vi "Dashboard Main1920x1080fixed_ALT.vi"() -> ()   [LabVIEW 2025]
uses:
  <vilib>/event_ctls.llb/eventvkey.ctl
  DashBoardGlobals.vi
  <vilib>/Rock Robotics/Network Tables/NT Read Numeric Array.vi
  <vilib>/Rock Robotics/WPI/Dashboard/WPI_DashboardLogging Global.vi
panel:
  in  "TCP":refnum<k5>
  out "NT Connection":bool
  out "Mode":T1(ring)=enum."Auto Disabled"
  out "BelowLeftCamBackground":bool
  out "Camera Perf":string
  in  "Rec Mode":enum32{"Stop", "Record", "Playback"}(radio)
  out "Robot IP":string
  in  "Dashboard Tab":T2(tab)
  out "MotorChart R":cluster{"Numeric":dbl, "Numeric":dbl}(graph)
  out "MotorChart L":cluster{"Numeric":dbl, "Numeric":dbl}(graph)
  out "MotorSliders R":cluster{"MotorSlide1":dbl, "MotorSlide2":dbl} {"MotorSlide2" scale=-1.0..1.0 scale format="%#_2e"; "MotorSlide1" scale=-1.0..1.0 scale format="%#_2e"}
  out "MotorSliders L":cluster{"MotorSlide1":dbl, "MotorSlide2":dbl} {"MotorSlide2" scale=-1.0..1.0 scale format="%#_2e"; "MotorSlide1" scale=-1.0..1.0 scale format="%#_2e"}
  out "JS1 Z":dbl(slide) scale=-1.0..1.0 scale format="%#_2e"
  out "JS1 Graph":cluster{"X":dbl, "Y":dbl}[](graph)
  out "JS1 Buttons":T3
  out "JS2 Z":dbl(slide) scale=-1.0..1.0 scale format="%#_2e"
  out "JS2 Graph":cluster{"X":dbl, "Y":dbl}[](graph)
  out "JS2 Buttons":T3
  out "Gyro":dbl(knob) scale=0.0..360.0
  in  "Update Agitator":bool
  in  "Agitator Desired Pct":dbl=1.0 min=-1.0 max=1.0 step=0.05 format="%8.2f"
  out "TurretLauncher/BallsLaunched":dbl caption="Balls Launched" format="%6.0f"
  out "Vision/Cam5Orientation":dbl caption="Cam 1 Yaw" format="%11.2f"
  out "Vision/Cam5Z":dbl caption="Cam 1 Z" format="%11.2f"
  out "Vision/Cam5Y":dbl caption="Cam 1 Y" format="%11.2f"
  out "Vision/Cam5Count":dbl caption="Cam1 Count" format="%13.0f"
  out "Vision/Cam5X":dbl caption="Cam 1 X" format="%11.2f"
  out "Vision/Cam4Orientation":dbl caption="Cam 1 Yaw" format="%11.2f"
  out "Vision/Cam4Z":dbl caption="Cam 1 Z" format="%11.2f"
  out "Vision/Cam4Y":dbl caption="Cam 1 Y" format="%11.2f"
  out "Vision/Cam4Count":dbl caption="Cam1 Count" format="%13.0f"
  out "Vision/Cam4X":dbl caption="Cam 1 X" format="%11.2f"
  out "Vision/Cam3Orientation":dbl caption="Cam 1 Yaw" format="%11.2f"
  out "Vision/Cam3Z":dbl caption="Cam 1 Z" format="%11.2f"
  out "Vision/Cam3Y":dbl caption="Cam 1 Y" format="%11.2f"
  out "Vision/Cam3Count":dbl caption="Cam1 Count" format="%13.0f"
  out "Vision/Cam3X":dbl caption="Cam 1 X" format="%11.2f"
  out "Vision/Cam2Orientation":dbl caption="Cam 1 Yaw" format="%11.2f"
  out "Vision/Cam2Z":dbl caption="Cam 1 Z" format="%11.2f"
  out "Vision/Cam2Y":dbl caption="Cam 1 Y" format="%11.2f"
  out "Vision/Cam2Count":dbl caption="Cam1 Count" format="%13.0f"
  out "Vision/Cam2X":dbl caption="Cam 1 X" format="%11.2f"
  out "Vision/Cam1Orientation":dbl caption="Cam 1 Yaw" format="%11.2f"
  out "Vision/Cam1Z":dbl caption="Cam 1 Z" format="%11.2f"
  out "Vision/Cam1Y":dbl caption="Cam 1 Y" format="%11.2f"
  out "Vision/Cam1Count":dbl caption="Cam1 Count" format="%13.0f"
  out "Vision/Cam1X":dbl caption="Cam 1 X" format="%11.2f"
  out "Climb/IsRetracted":bool caption="Retracted"
  out "Climb/MotorDemand":dbl caption="Pos Motor Dmd" format="%11.2f"
  out "Climb/Position":dbl caption="Position Act" format="%12.1f"
  out "Climb/RetractedLimitSwitch":bool caption="Retract Limit Switch"
  out "Climb/IsExtended":bool caption="Extended"
  out "AgitatorSystem/AgitatorStalled":bool caption="Agitator Stalled"
  out "AgitatorSystem/AgitatorRPMTarget":dbl caption="Speed Dmd  RPM" format="%12.1f"
  out "AgitatorSystem/AgitatorRPM":dbl caption="Speed  RPM" format="%12.1f"
  out "AgitatorSystem/AgitatorOutput":dbl caption="Motor Dmd" format="%11.2f"
  out "AgitatorSystem/AgitatorState":bool caption="Agitator On"
  out "IntakeSystem/BallMotorStalled":bool caption="Ball Intake Stalled"
  out "IntakeSystem/BallIntakeOn":bool caption="Ball Intake On"
  out "IntakeSystem/IntakeMotorRPM":dbl caption="Intake RPM" format="%12.1f"
  out "IntakeSystem/IntakeMotorOut":dbl caption="Intake Motor Dmd" format="%11.2f"
  out "TurretLauncher/TurretAngleVelocityDegSec":dbl caption="Pos Rate Deg/Sec" format="%12.1f"
  out "TurretLauncher/TurretManualMode":bool caption="Manual"
  out "TurretLauncher/TurretEncoderRotation":dbl caption="Pos Deg" format="%12.1f"
  out "TurretLauncher/TurretPositionOnTarget":bool caption="On Target"
  out "TurretLauncher/TurretMotorDmd":dbl caption="Motor Output" format="%11.2f"
  out "TurretLauncher/TurretDesiredAngle":dbl caption="Pos Dmd Deg" format="%12.1f"
  out "TurretLauncher/TurretclockwiseLimitSwitch":bool caption="CW Limit"
  out "TurretLauncher/TurretcounterclockwiseLimitSwitch":bool caption="CCW Limit"
  out "TurretLauncher/TurretDesiredAngleVel":dbl caption="Angle Velocity" format="%11.2f"
  out "TurretLauncher/TargetAngle":dbl caption="Angle" format="%11.2f"
  out "TurretLauncher/TargetDistance":dbl caption="Distance" format="%11.2f"
  out "FeederSystem/FeederTargetRPM":dbl caption="Speed Dnd RPM" format="%12.0f"
  out "FeederSystem/FeederRPM":dbl caption="Speed RPM" format="%12.0f"
  out "FeederSystem/FeederOutput":dbl caption="Motor Dmd" format="%11.2f"
  out "FeederSystem/FeederState":bool caption="Feeder On"
  out "MatchSystem/RobotCodePhase":T4(ring) caption="Code Phase"
  out "MatchSystem/isRed":bool caption="Is Red"
  out "MatchSystem/isBlue":bool caption="Is Blue"
  out "Supervisory/Mode":string caption="Mode"
  out "IntakeSystem/IntakeAngleMotorOut":dbl caption="Pos Motor Dmd" format="%11.2f"
  out "IntakeSystem/IntakeAngleTarget":dbl caption="Position Dmd Deg" format="%12.1f"
  out "IntakeSystem/IntakeAngleActual":dbl caption="Position Act Deg" format="%12.1f"
  out "IntakeSystem/IntakeLimitIsPressed":bool caption="LowLimitSwitch"
  out "IntakeSystem/IntakeIsExtended":bool caption="Extended"
  out "TurretLauncher/LauncherOn":bool caption="Launcher On"
  out "TurretLauncher/LauncherManualMode":bool caption="Manual"
  out "TurretLauncher/LauncherSpeed2":dbl caption="Motor 2 Speed" format="%11.0f"
  out "TurretLauncher/LauncherSpeed1":dbl caption="Motor 1 Speed" format="%11.0f"
  out "TurretLauncher/LauncherSpeedActual":dbl caption="Average Speed RPM" format="%11.0f"
  out "TurretLauncher/LauncherMotorDmd":dbl caption="Motor Dmd" format="%11.2f"
  out "TurretLauncher/LauncherTargetSpeed":dbl caption="Desired Speed RPM" format="%11.0f"
  out "TurretLauncher/LauncherSpeedOnTarget":bool caption="On Target"
  out "Teleop/GoClimb":bool caption="GO CLIMB"
  out "Teleop/FieldOriented":bool caption="Field Oriented"
  out "AutoSystem/StepTime":dbl caption="Step Time" format="%11.2f"
  out "Auto Selector":string caption="Name"
  out "AutoSystem/Step":T5(ring) caption="Cmd Name"
  out "AutoSystem/function":string caption="Function"
  out "AutoSystem/Parm2":dbl caption="Parm 2" format="%11.2f"
  out "AutoSystem/Parm1":dbl caption="Parm 1" format="%11.2f"
  out "AutoSystem/Timeout":dbl caption="Time out Sec" format="%11.2f"
  out "AutoSystem/Parm3":dbl caption="Parm 3" format="%11.2f"
  out "AutoSystem/Step":dbl caption="Cmd" format="%13.0f"
  out "TrajectorySystem/done":bool caption="Done"
  out "TrajectorySystem/ElapsedTrajTime":dbl caption="Elapsed Time" format="%12.1f"
  out "TrajectorySystem/rotErr":dbl caption="Rotational Error" format="%11.2f"
  out "TrajectorySystem/yErr":dbl caption="Y Error" format="%11.2f"
  out "TrajectorySystem/timeLengthOfTrajectory":dbl caption="Total Time" format="%12.1f"
  out "TrajectorySystem/xErr":dbl caption="X Error" format="%11.2f"
  out "TrajectorySystem/onTarget":bool caption="On Target"
  out "SwerveDrive/omegaActual":dbl caption="Vel Rot" format="%11.2f"
  out "SwerveDrive/vyActual":dbl caption="Vel Y" format="%12.1f"
  out "SwerveDrive/vyTarget":dbl caption="Vel Y Dmd" format="%12.1f"
  out "SwerveDrive/vxActual":dbl caption="Vel X" format="%12.1f"
  out "SwerveDrive/vxTarget":dbl caption="Vel X Dmd" format="%12.1f"
  out "SwerveDrive/GyroYaw":dbl caption="Gyro Yaw" format="%12.1f"
  out "SwerveDrive/GyroRoll":dbl caption="Gyro Roll" format="%12.1f"
  out "SwerveDrive/omegaTarget":dbl caption="Vel Rot Dmd" format="%11.2f"
  out "SwerveDrive/GyroPitch":dbl caption="Gyro Pitch" format="%12.1f"
  out "SwerveDrive/GyroConnected":bool caption="Gyro Connected"
  in  "Select Auto":string(combo)="Select Autonomous ..."
  out "Odometry/Rotation_position":dbl caption="Rotation Rad" format="%11.2f"
  out "Odometry/Y_position":dbl caption="Y Pos M" format="%11.2f"
  out "Odometry/execElapsedTime":dbl caption="Elapsed Time" format="%9.3f"
  out "Odometry/X_position":dbl caption="X Pos M" format="%11.2f"
  in  "Test Slider":dbl(slide) scale=0.0..100.0 scale format="%#_3g"
  in  "On/Off":bool caption="Solenoid"
  in  "Test Name":u16(ring) items=["Select the test to run..."]
  in  "Test Tree":string(tree)
  in  "Motor":cluster{"Value":dbl, "Enable":bool} {"Value" scale=-1.0..1.0 scale format="%#_3g"}
  out "Progress":T6 {"Test Progress" scale=0.0..100.0}
  in  "Rev/Fwd":cluster{"Forward":bool, "Reverse":bool}
  in  "Test Ring":u16(ring) items=["Monochrome", "Color"]
  in  "CheckList":i32(listbox)
  out "Tree":string(tree)
  out "Background":bool
  # "Drive Motors"
  # "Front"
  # "Right"
  # "Left"
  # "Back"
  # "Joysticks"
  # "TARGET"
  # "BALLS LAUNCHED"
  # "VISION"
  # "Cam 1"
  # "Cam 2"
  # "Cam 3"
  # "Cam 4"
  # "Cam 5"
  # "Count"
  # "X"
  # "Y"
  # "Z"
  # "Yaw"
  # "CLIMB"
  # "AGITATOR"
  # "BALL INTAKE"
  # "TURRET"
  # "FEEDER"
  # "MATCH"
  # "SUPERVISORY"
  # "INTAKE ARM"
  # "LAUNCHER"
  # "TELEOP"
  # "AUTO"
  # "TRAJECTORY"
  # "DRIVE"
  # "ODOMETRY"
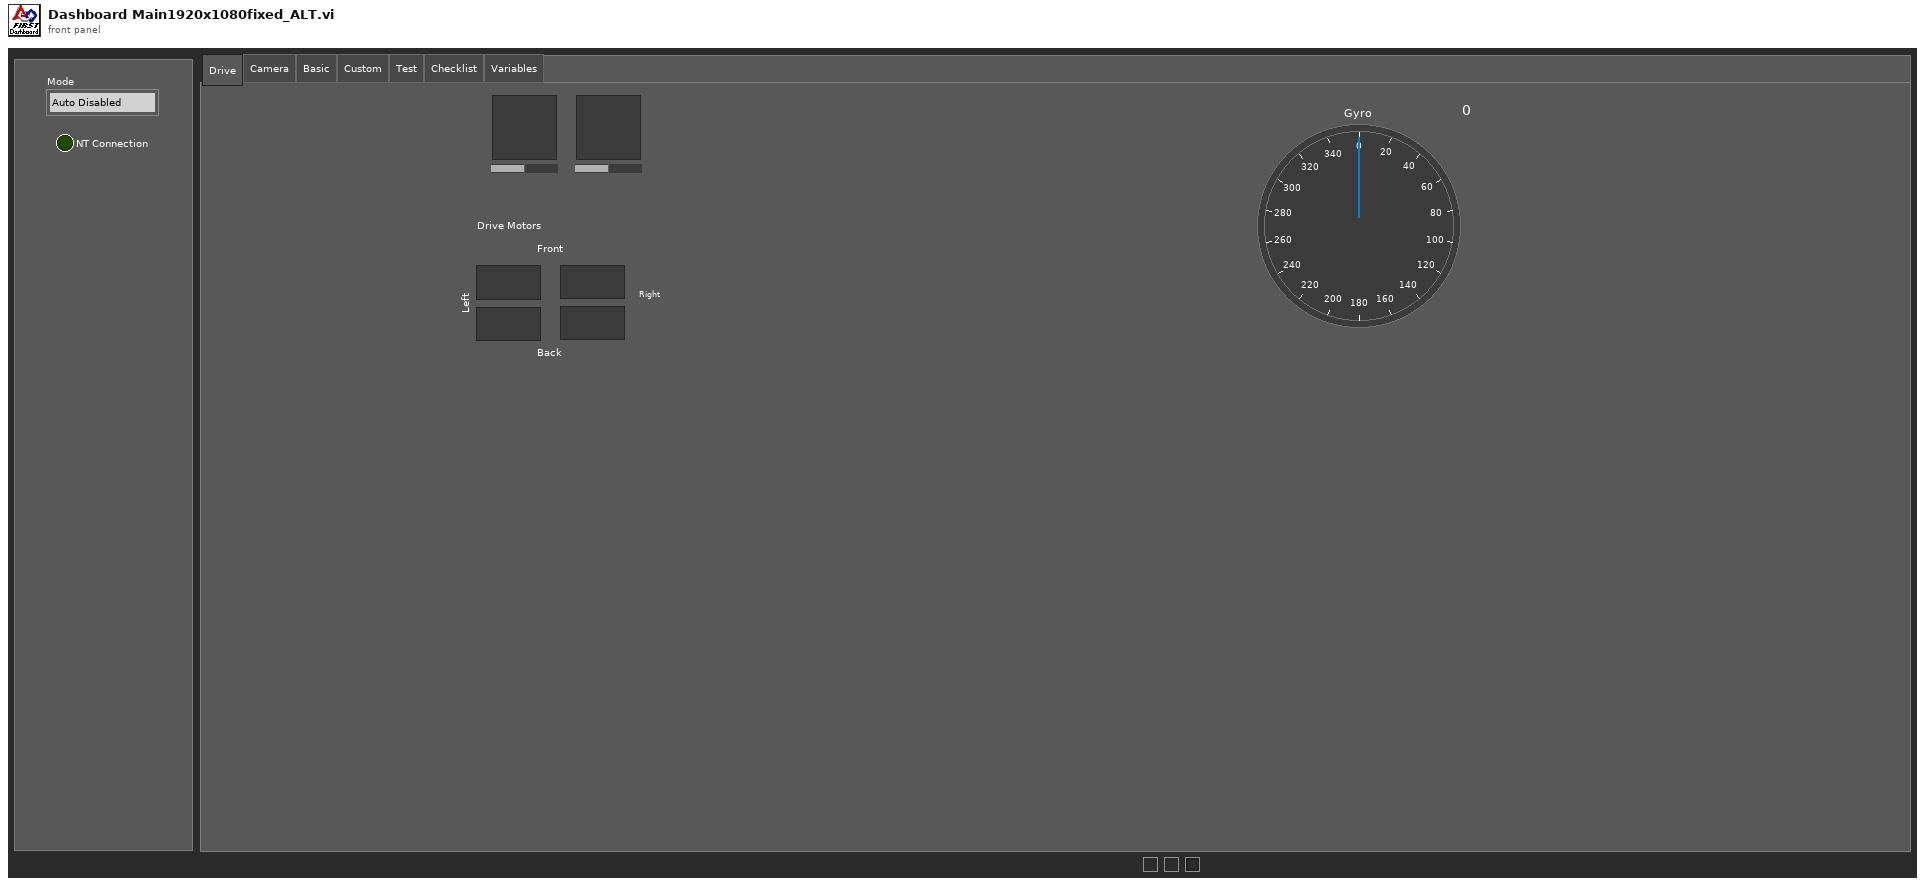
[diagram p1: front panel]
types:
  T1 = enum8{"Tele-Op Disabled", "Tele-Op Enabled", "Auto Disabled", "Auto Enabled", "Test Disabled", "Test Enabled", "Disconnected", "No Code", "E-Stop"}
  T2 = enum32{"Drive", "Camera", "Basic", "Custom", "Test", "Checklist", "Variables"}
  T3 = cluster{bool, bool, bool, bool, bool, bool, bool, bool, bool, bool, bool, bool}
  T4 = enum16{"Initial Startup", "Gyro Calibrated", "Trajectories Read", "Autos Read", "Startup Done", "Exec Disable Code", "Auto Init Done", "Auto Running", "Teleop Running"}
  T5 = enum16{"Drive Straight", "Drive Spin", "Follow Abs Traj", "Follow Rel Traj", "Wait", "Follow Abs Traj w/Event", "Follow Rel Traj w/Event", "Collect", "Shoot", "Balls To Alliance", "Climb", "Descend", "Unknown"}
  T6 = cluster{"Test Progress":u8, "Test Progress Text":string}
  T7 = enum32{"Invalid", "Standard", "Closed", "Hidden", "Minimized", "Maximized"}
  T8 = enum32{"Drive", "Camera", "Basic", "Custom", "Test", "Commands", "Checklist", "Variables"}
  T9 = cluster{"Error Strings":string, "Disable Counts":cluster{u16, u16}, "Rail Faults":cluster{u16, u16, u16}, "Robot IP":string, "DB Mode":u8, "Event Info":cluster{"Name":string, "Type":u8, "Number":u16, "Replay":u8}}
  T10 = cluster{"Storage":cluster{"Disk Free":u64, "RAM Block":u32, "RAM free":u32}, "CPU Utilization":cluster{"CPU % ISR":sgl, "CPU % Time Crit":sgl, "CPU % Timed Str":sgl, "CPU % High":sgl, "CPU % Above":sgl, "CPU % Normal":sgl, "CPU % Low":sgl}, "CAN":cluster{"% Bus Utilization":sgl, "Bus Off Cnt":u32, "TX_FIFO Full Cnt":u32, "Receive Error Cnt":u8, "Transmit Error Cnt":u8}, "HID":cluster{"HID Outputs":u32, "Rumble Low":u16, "Rumble High":u16}[]}
  T11 = cluster{"Status bits":cluster{"Test Mode":bool, "Autonomous":bool, "Enabled":bool, "Code Start":bool, "Brownout":bool, "Reserved 2":bool, "Reserved 3":bool, "E-Stop":bool}, "Code Trace":cluster{"Disabled":bool, "TeleOp":bool, "Auto":bool, "Test":bool}, "Controller Type":enum16{"unknown", "cRIO", "roboRio"}, "Code?":enum16{"unknown", "noCode", "code"}, "Battery V":dbl}
  T12 = cluster{"Control Bits":cluster{"TestMode":bool, "Autonomous":bool, "Enabled":bool, "FMS Present":bool, bool, bool, bool, "E-Stop":bool}, "Team Station ":u8, "Countdown":sgl, "Joystick Values":cluster{"Axes":dbl[], "Buttons":bool[], "POVs":i16[]}[]}
  T13 = cluster{"Axes":dbl[], "Buttons":bool[], "POVs":i16[]}[]
  T14 = cluster{"Axes":dbl[], "Buttons":bool[], "POVs":i16[]}
  T15 = cluster{"Buttons[0]":bool, "Buttons[1]":bool, "Buttons[2]":bool, "Buttons[3]":bool, "Buttons[4]":bool, "Buttons[5]":bool, "Buttons[6]":bool, "Buttons[7]":bool, "Buttons[8]":bool, "Buttons[9]":bool, "Buttons[10]":bool, "Buttons[11]":bool}
  T16 = cluster{"Dashboard Tab":refnum<vi>, "Background":refnum<vi>, "Rec Mode":refnum<vi>, "Test Slider":refnum<vi>, "On/Off ":refnum<vi>, "Test Ring":refnum<vi>, "Rev/Fwd":refnum<vi>, "Test Name":refnum<vi>, "Motor":refnum<vi>, "Progress":refnum<vi>, "CheckList":refnum<vi>, "Tree":refnum<vi>, "Test Tree":refnum<vi>, "Camera Perf":refnum<vi>}
  T17 = cluster{"Operation":enum16{"Update", "Clear"}, "Color Box":u32}[]
  T18 = typedef "eventvkey.ctl" = enum16{"ASCII", "Enter", "Return", "Shift", "Ctrl", "Alt", "Cmd", "Opt", "Caps", "NumLock", "Clear", "Break", "Up", "Down", "Left", "Right", "Insert", "Delete", "Home", "End", "PageUp", "PageDown", "Escape", "Help", "Pause", "ScrollLock", "F1", "F2", "F3", "F4", "F5", "F6", "F7", "F8", "F9", "F10", "F11", "F12", "F13", "F14", "F15", "F16", "F17", "F18", "F19", "F20", "F21", "F22", "F23", "F24", "Play", "VolumeUp", "VolumeDown", "Mute", "Two Byte Char"}
  T19 = cluster{"Image Size":bool, "Image Type":bool, "Pixel Value":bool, "ROI Information":bool, "Zoom Factor":bool}
  T20 = cluster{"Operation":enum16{"Update", "Clear"}, "Color Box":u32}
  T21 = cluster{"Shift":bool, "Ctrl":bool, "Alt":bool, "Cmd":bool, "Opt":bool}
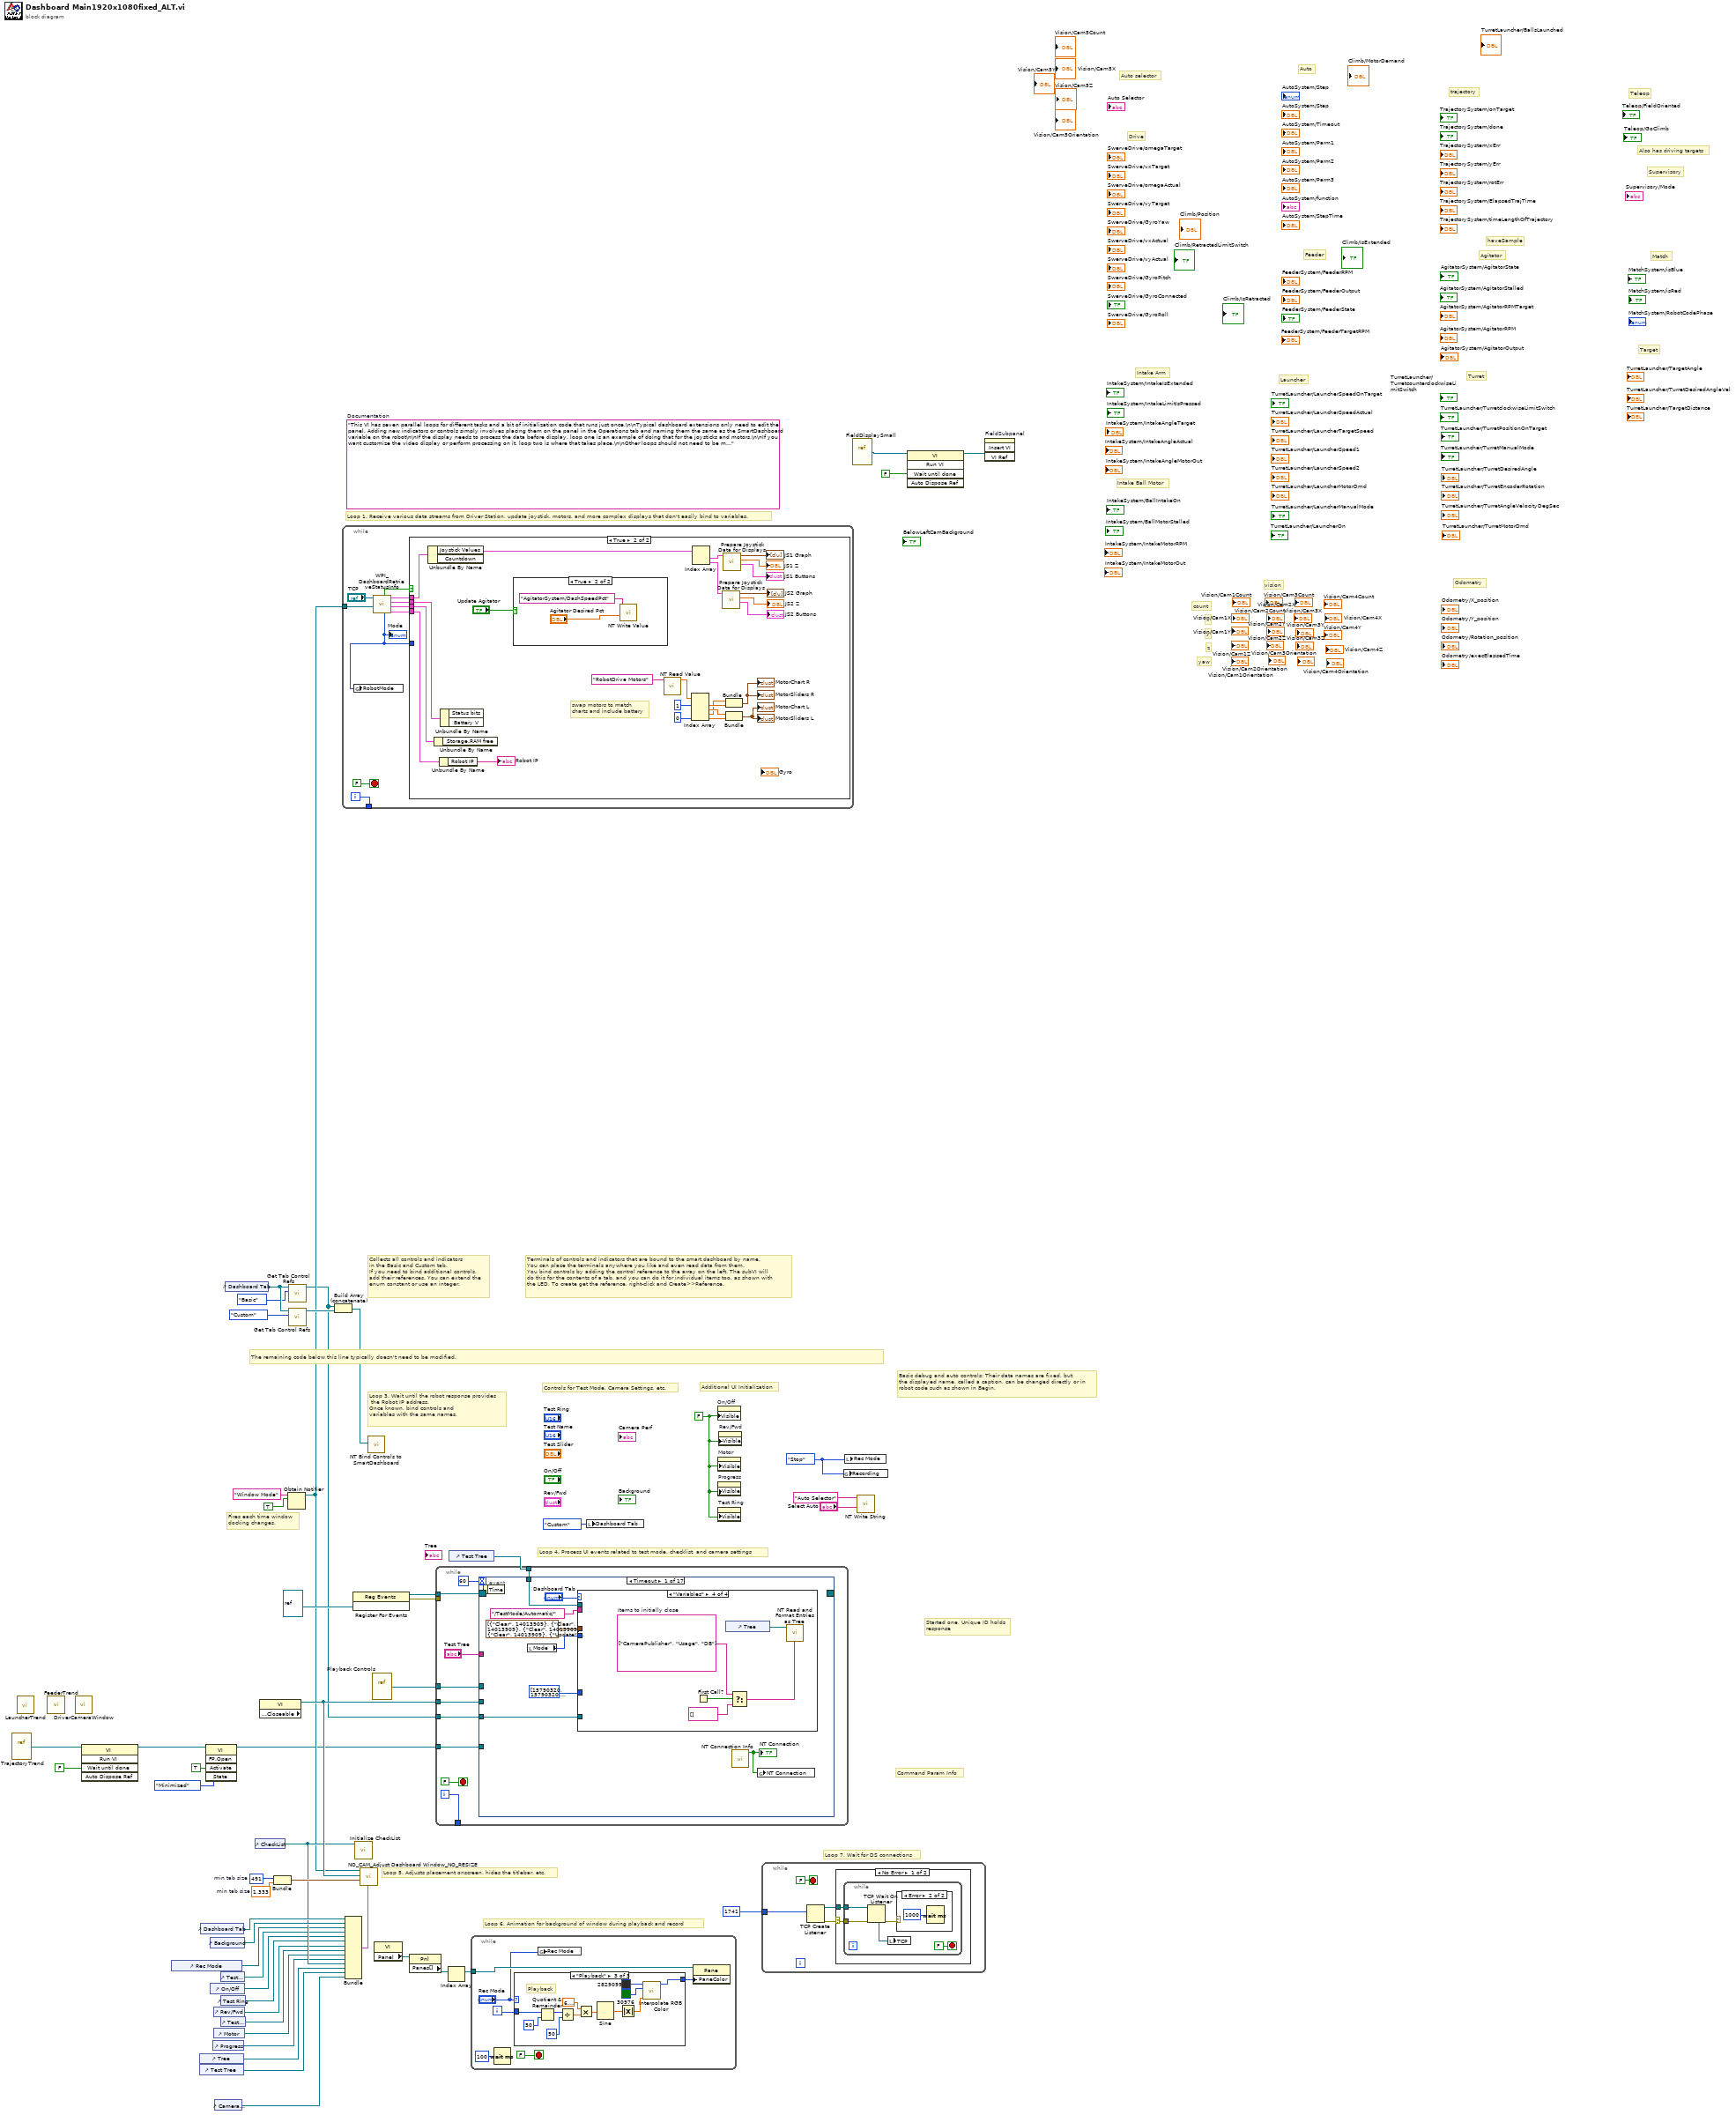
[diagram p0: block diagram]
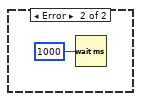
[diagram p3: hidden frame]
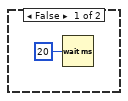
[diagram p4: hidden frame]
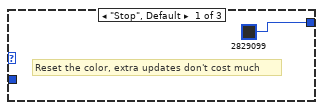
[diagram p6: hidden frame]
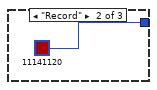
[diagram p7: hidden frame]
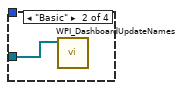
[diagram p9: hidden frame]
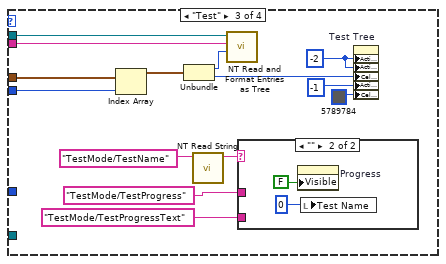
[diagram p10: hidden frame]
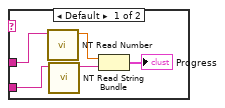
[diagram p11: hidden frame]
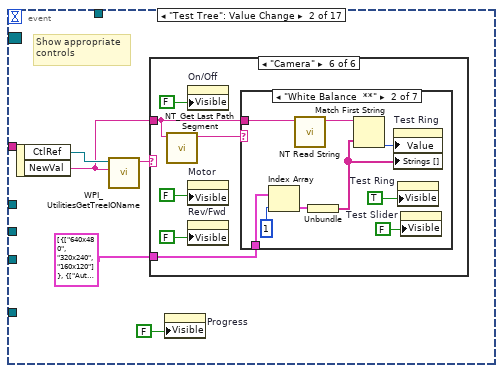
[diagram p12: hidden frame]
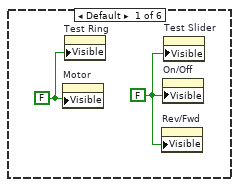
[diagram p13: hidden frame]
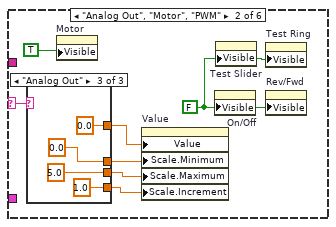
[diagram p14: hidden frame]
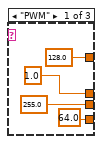
[diagram p15: hidden frame]
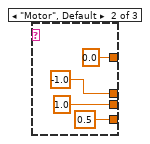
[diagram p16: hidden frame]
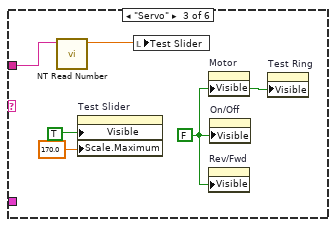
[diagram p17: hidden frame]
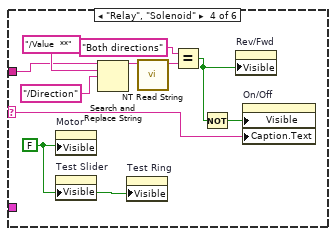
[diagram p18: hidden frame]
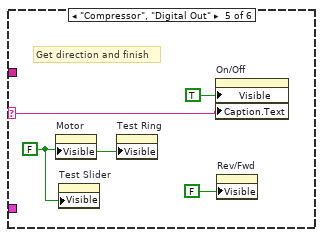
[diagram p19: hidden frame]
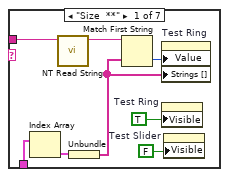
[diagram p20: hidden frame]
diagram:
  w35 = 491  # min tab size
  w34 = 1.333  # min tab size
  w41 = enum32{"Stop", "Record", "Playback"}."Stop" ("Rec Mode")
  w19 = FALSE ("Visible")
  (unwired) "This VI has seven parallel loops for different tasks and a bit of initialization code that runs just once.\n\nTypical dashboard extensions only need to edit the panel. Adding new indicators or controls simply involves placing them on the panel in the Operations tab and naming them the same as the SmartDashboard variable on the robot\n\nIf the display needs to process the data before display, loop one is an example of doing that for the joysticks and motors.\n\nIf you want customize the video display or perform processing on it, loop two is where that takes place.\n\nOther loops should not need to be modified. They are pretty standard, and document the task they perform."  # Documentation
  # "Intake Ball Motor"
  # "Target"
  # "Match"
  # "Supervisory"
  # "haveSample"
  # "Also has driving targets"
  # "Teleop"
  # "Odometry"
  # "Auto selector"
  # "Drive"
  # "Auto"
  # "trajectory"
  # "Feeder"
  # "Agitator"
  # "Intake Arm"
  # "Turret"
  # "yaw"
  # "z"
  # "y"
  # "x"
  # "count"
  # "vision"
  # "Launcher"
  # "Command Param Info"
  # "Started one, Unique ID holds\nresponse"
  # "Loop 7. Wait for DS connections"
  # "Basic debug and auto controls: Their data names are fixed, but\nthe displayed name, called a caption, can be changed directly or in\nrobot code such as shown in Begin."
  # "Controls for Test Mode, Camera Settings, etc."
  # "Additional UI Initialization"
  # "Loop 6. Animation for background of window during playback and record"
  # "Fires each time window\ndocking changes."
  # "Collects all controls and indicators\nin the Basic and Custom tab.\nIf you need to bind additional controls,\nadd their references. You can extend the\nenum constant or use an integer."
  # "The remaining code below this line typically doesn't need to be modified."
  # "Loop 4. Process UI events related to test mode, checklist, and camera settings"
  # "Terminals of controls and indicators that are bound to the smart dashboard by name.\nYou can place the terminals anywhere you like and even read data from them.\nYou bind controls by adding the control reference to the array on the left. The subVI will\ndo this for the contents of a tab, and you can do it for individual items too, as shown with\nthe LED. To create get the reference, right-click and Create>>Reference."
  # "Loop 3. Wait until the robot response provides\n the Robot IP address.\nOnce known, bind controls and\nvariables with the same names."
  # "Loop 5. Adjusts placement onscreen, hides the titlebar, etc."
  # "Loop 1. Receive various data streams from Driver Station, update joystick, motors, and more complex displays that don't easily bind to variables."
  n1 = vi-ref "TrajectoryTrend.vi"() -> (w5:refnum<vi>)
  n2 = call "LauncherTrend.vi"() -> ()  [unwired: 12 in]
  n3 = call "FeederTrend.vi"() -> ()  [unwired: 12 in]
  n4 = call "DriverCameraWindow.vi"() -> ()  [unwired: 1 in]
  n5 = invoke class="VI" method="Run VI"(reference=w5, "Wait until done"=FALSE ("Wait Until Done")) -> (reference out=w4:refnum<vi>)  [unwired: 3 in, 4 out]
  n6 = control-ref of="Rec Mode"() -> (w25:refnum<vi>)
  n7 = control-ref of="Tree"() -> (w29:refnum<vi>)
  n8 = control-ref of="Test Tree"() -> (w28:refnum<vi>)
  n9 = control-ref of="Dashboard Tab"() -> (w36:refnum<vi>)
  n10 = invoke class="VI" method="FP.Open"(reference=w4, "Activate"=TRUE ("Activate?"), "State"=T7."Minimized") -> (reference out=w1:refnum<vi>)  [unwired: 2 in, 4 out]
  n11 = control-ref of="Background"() -> (w32:refnum<vi>)
  n12 = control-ref of="On/Off"() -> (w23:refnum<vi>)
  n13 = control-ref of="Progress"() -> (w20:refnum<vi>)
  n14 = control-ref of="Rev/Fwd"() -> (w21:refnum<vi>)
  n15 = control-ref of="Motor"() -> (w26:refnum<vi>)
  n16 = control-ref of="Camera Perf"() -> (w16:refnum<vi>)
  n17 = control-ref of="Test Slider"() -> (w24:refnum<vi>)
  n18 = control-ref of="Test Ring"() -> (w22:refnum<vi>)
  n19 = control-ref of="Test Name"() -> (w27:refnum<vi>)
  n20 = control-ref of="Dashboard Tab"() -> (w39:refnum<vi>)
  n21 = control-ref of="CheckList"() -> (w30:refnum<vi>)
  n22 = property class="VI" props=["Front Panel.Closeable"]() -> (reference out=w40:refnum<vi>)  [unwired: 2 in, 2 out]
  n23 = Bundle("min tab size"=w35, "min tab size"=w34) -> (w33:cluster{"min tab size":i32, "min tab size":dbl})  [unwired: 1 in]
  n24 = Obtain Notifier(name (unnamed)="Window Mode", notification data type=TRUE) -> (notifier out=w18:refnum<notifier>)  [unwired: 2 in, 2 out]
  n25 = call <vilib>:"Get Tab Control Refs.vi"("Page Index"=T8."Basic" ("Dashboard Tab"), "TabControl in"=w39) -> ("ControlsOnPage"=w15:refnum<vi>[])  [unwired: 9 in]
  n26 = call <vilib>:"Get Tab Control Refs.vi"("Page Index"=T8."Custom" ("Dashboard Tab"), "TabControl in"=w39) -> ("ControlsOnPage"=w38:refnum<vi>[])  [unwired: 9 in]
  n27 = Build Array (concatenate)(w15, w38) -> (w37:refnum<vi>[])
  n28 = while {
    tunnel: [w60] -> _
    tunnel: w18 -> [w53]
    i -> [w60]
    stop <- FALSE stop-if-true
    n29 = call <vilib>:"WPI_DashboardRetrieveStatusInfo.vi"("Window Mode Notifier"=w53, "TCP Cnx"="TCP") -> ("Power and Errors"=w55:T9, "Robot Metrics"=w58:T10, "Status Info"=w59:T11, "Control Info"=w56:T12, "Robot Mode"=w52:T1, "Process?"=w57:bool)  [unwired: 4 in]
    "Mode" <- w52
    n30 = global write "DashBoardGlobals.vi" "RobotMode"(w52) -> ()
    n31 = case shown="True" w57 {
      tunnel: w59 -> [_ w87]
      tunnel: w58 -> [_ w86]
      tunnel: w56 -> [_ w85]
      tunnel: w55 -> [_ w84]
      tunnel: w52 -> [_ _]
      frame False {
        n32 = Wait (ms)(milliseconds to wait=u32 20) -> ()  [unwired: 1 out]
      }
      frame True {
        # "swap motors to match\ncharts and include battery"
        n33 = Unbundle By Name(w85) -> ("Joystick Values"=w75:T13)  [unwired: 1 out]
        n34 = Unbundle By Name(w86) -> ()  [unwired: 1 out]
        n35 = Unbundle By Name(w84) -> ("Robot IP"=→"Robot IP":string)
        n36 = Unbundle By Name(w87) -> ()  [unwired: 2 out]
        n37 = case shown="True" "Update Agitator" {
          frame False {
          }
          frame True {
            n38 = call-poly <vilib>:"NT Write Value.vi"("value"="Agitator Desired Pct", "name"="AgitatorSystem/DashSpeedPct") -> ()  [unwired: 9 in, 1 out]
          }
        }
        n39 = call-poly <vilib>:"NT Read Value.vi"("name"="RobotDrive Motors" ("Name")) -> ("value"=w65:dbl[])  [unwired: 8 in, 2 out]
        n40 = Index Array(array=w65, index #1=1, index #4=0) -> (element #1=w79:dbl, element #2=w80:dbl, element #3=w78:dbl, element #4=w83:dbl)  [unwired: 2 in]
        n41 = Index Array(array=w75) -> (element #1=w74:T14, element #2=w70:T14)  [unwired: 2 in]
        n42 = call "Prepare Joystick Data for Displays.vi"("Joystick Values"=w70) -> ("Buttons"=→"JS2 Buttons":T15, "Z Axis"=→"JS2 Z":dbl, "Cartesian Data"=→"JS2 Graph":cluster{"X axis":dbl, "X axis":dbl}[])  [unwired: 8 in]
        n43 = call "Prepare Joystick Data for Displays.vi"("Joystick Values"=w74) -> ("Buttons"=→"JS1 Buttons":T15, "Z Axis"=→"JS1 Z":dbl, "Cartesian Data"=→"JS1 Graph":cluster{"X axis":dbl, "X axis":dbl}[])  [unwired: 8 in]
        n44 = Bundle("Numeric"=w78, "Numeric"=w79) -> (→"MotorChart R" →"MotorSliders R":cluster{"Numeric":dbl, "Numeric":dbl})  [unwired: 1 in]
        n45 = Bundle("Numeric"=w80, "Numeric"=w83) -> (→"MotorChart L" →"MotorSliders L":cluster{"Numeric":dbl, "Numeric":dbl})  [unwired: 1 in]
      }
    }
  }
  n46 = Bundle("Dashboard Tab"=w36, "Background"=w32, "Rec Mode"=w25, "Test Slider"=w24, "On/Off"=w23, "Test Ring"=w22, "Rev/Fwd"=w21, "Test Name"=w27, "Motor"=w26, "Progress"=w20, "CheckList"=w30, "Tree"=w29, "Test Tree"=w28, "Camera Perf"=w16) -> (w31:T16)  [unwired: 1 in]
  n47 = register-events(refnum<vi> refnum) -> (reference out=w44:refnum<event-registration>, error out=w43:errorcluster)  [unwired: 2 in]
  n48 = call "Initialize CheckList.vi"("ListBox in"=w30) -> ()  [unwired: 11 in]
  n49 = call "NO_CAM_Adjust Dashboard Window_NO_RESIZE.vi"("Sizing Refnums"=w31, "Size Constraints"=w33, "VI"=w40, "WIn Mode"=w18) -> ()  [unwired: 8 in]
  n50 = call <vilib>:"NT Bind Controls to SmartDashboard.vi"("Bound Control Refs"=w37) -> ()  [unwired: 11 in]
  n51 = vi-ref "Playback Controls.vi"() -> (w45:refnum<vi>)
  n52 = property class="VI"() -> ("Panel"=w47:refnum<vi>)  [unwired: 2 in, 2 out]
  n53 = property class="Pnl"(reference=w47) -> ("Panes[]"=w48:refnum<vi>[])  [unwired: 1 in, 2 out]
  n54 = Index Array(array=w48) -> (element=w46:refnum<vi>)  [unwired: 1 in]
  n55 = control-ref of="Test Tree"() -> (w49:refnum<vi>)
  n56 = while {
    tunnel: [w96] -> _
    tunnel: w49 -> [w95]
    tunnel: w45 -> [w94]
    tunnel: w44 -> [w93]
    tunnel: w43 -> [_]
    tunnel: w40 -> [w92]
    tunnel: w15 -> [w91]
    tunnel: w1 -> [w90]
    i -> [w96]
    stop <- FALSE stop-if-true
    n57 = event shown="[0] Timeout" {
      selector: w93 -> [_ _ _ _ _ _ _ _ _ _ _ _ _ _ _ _ _]
      dyn-events: [_ _ _ _ _ _ _ _ _ _ _ _ _ w299 _ _ _] -> _
      timeout: u32 60 ("milliseconds to wait") -> [_ _ _ _ _ _ _ _ _ _ _ _ _ _ _ _ _]
      tunnel: w95 -> [w107 _ _ _ _ _ _ _ _ _ _ _ _ _ _ _ _]
      tunnel: "Test Tree" -> [_ _ _ _ _ _ _ _ w274 w281 w282 w285 w292 _ _ _ _]
      tunnel: w94 -> [_ _ _ _ _ _ _ _ _ _ _ _ _ w301 _ w319 _]
      tunnel: w92 -> [_ _ _ _ _ _ _ _ _ _ _ _ _ w297 _ _ _]
      tunnel: w91 -> [w102 _ _ _ _ _ _ _ _ _ _ _ _ _ _ _ _]
      tunnel: w90 -> [_ _ _ _ _ _ _ _ _ _ _ _ _ _ _ w314 _]
      event Timeout {
        n58 = event-data() -> ()  [unwired: 1 in, 1 out]
        n59 = local read "Mode"() -> (w105:T1)
        n60 = case shown="\"Variables\"" "Dashboard Tab" {
          tunnel: w107 -> [_ _ w122 _]
          tunnel: "/TestMode/Automatic/" ("Name Pattern") -> [_ _ w121 _]
          tunnel: T17 [{"Operation"=enum."Clear", "Color Box"=14013909}, {"Operation"=enum."Clear", "Color Box"=14013909}, {"Operation"=enum."Clear", "Color Box"=14013909}, {"Operation"=enum."Clear", "Color Box"=14013909}, {"Operation"=enum."Update", "Color Box"=14013909}, {"Operation"=enum."Update", "Color Box"=16777215}, {"Operation"=enum."Clear", "Color Box"=14013909}, {"Operation"=enum."Clear", "Color Box"=14013909}, {"Operation"=enum."Clear", "Color Box"=14013909}] -> [_ _ w114 _]
          tunnel: w105 -> [_ _ w113 _]
          tunnel: u32[] [15790320, 15790320, 15790320, 15790320, 16777215, 16777215, 15790320, 15790320, 15790320] -> [_ _ _ _]
          tunnel: w102 -> [_ w108 _ _]
          frame "Custom", Default {
          }
          frame "Basic" {
            n61 = call <vilib>:"WPI_DashboardUpdateNames.vi"("Controls on Tab"=w108) -> ()  [unwired: 11 in]
          }
          frame "Test" {
            w120 = -2 ("Active Item:Row Number")
            n62 = Index Array(array=w114, index=w113) -> (element=w115:T20)
            n63 = Unbundle(w115) -> ("Operation"=w116:enum16{"Update", "Clear"}, "Color Box"=w117:u32)
            n64 = call <vilib>:"NT Read String.vi"("name"="TestMode/TestName" ("Name")) -> ("value"=w111:string)  [unwired: 8 in, 2 out]
            n65 = call <vilib>:"NT Read and Format Entries as Tree.vi"("Operation"=w116, "Name Pattern"=w121, "Tree Refnum"=w122) -> ()  [unwired: 7 in, 2 out]
            n66 = case shown="\"\"" w111 {
              tunnel: "TestMode/TestProgress" ("Name") -> [w124 _]
              tunnel: "TestMode/TestProgressText" ("Name") -> [w123 _]
              frame Default {
                n67 = call <vilib>:"NT Read Number.vi"("name"=w124) -> ("value"=w125:dbl)  [unwired: 8 in, 2 out]
                n68 = call <vilib>:"NT Read String.vi"("name"=w123) -> ("value"=w126:string)  [unwired: 8 in, 2 out]
                n69 = Bundle("value"=w125, "value"=w126) -> (→"Progress":cluster{"value":dbl, "value":string})  [unwired: 1 in]
              }
              frame "" {
                n70 = property on="Progress" class="Clust (strict)"("Visible"=FALSE) -> ()  [unwired: 2 in, 2 out]
                n71 = local write "Test Name"(u16 0) -> ()
              }
            }
            n72 = property on="Test Tree" class="Tree (strict)"("Active Item Row Number"=w120, "ActiveColNum"=w120, "CellBG"=w117, "Active Item Row Number"=-1 ("Active Item:Row Number"), "CellBG"=u32 5789784 ("Color Box")) -> ()  [unwired: 2 in, 2 out]
          }
          frame "Variables" {
            w132 = string[] ["CameraPublisher", "Usage", "DB"]  # Items to initially close
            n73 = First Call?() -> (First Call?: T/F=w133:bool)
            n74 = control-ref of="Tree"() -> (w134:refnum<vi>)
            n75 = Select(t=w132, s=w133, f=string[] []) -> (s? t:f=w130:string[])
            n76 = call <vilib>:"NT Read and Format Entries as Tree.vi"("Tags to  Close"=w130, "Tree Refnum"=w134) -> ()  [unwired: 8 in, 2 out]
          }
        }
        n77 = call <vilib>:"NT Connection Info.vi"() -> ("Connected"=w100:bool)  [unwired: 11 in]
        "NT Connection" <- w100
        n78 = global write "DashBoardGlobals.vi" "NT Connection"(w100) -> ()
      }
      event "Test Tree": Value Change {
        # "Show appropriate\ncontrols"
        n79 = event-data() -> ("CtlRef"=w138:refnum<vi>, "NewVal"=w136:string)  [unwired: 1 in]
        n80 = call <vilib>:"WPI_UtilitiesGetTreeIOName.vi"("NewVal"=w136, "TreeControl in"=w138) -> ("I/O Name"=w139:string)  [unwired: 9 in]
        n81 = case shown="\"Camera\"" w139 {
          selector: w139 -> [_ w146 _ w168 w177 _]
          tunnel: w136 -> [_ _ w165 w167 _ w184]
          tunnel: cluster{string[]}[] [{["640x480", "320x240", "160x120"]}, {["Auto", "Fixed indoor", "Fixed outdoor 1", "Fixed outdoor 2", "Fixed fluorescent 1", "Fixed fluorescent 2", "Hold current"]}, {["Auto", "Flicker-free 50 Hz", "Flicker-free 60 Hz", "Hold current"]}, {["None", "Prioritize frame rate", "Prioritize image quality"]}, {["Monochrome", "Color"]}] -> [_ _ _ _ _ w183]
          frame Default {
            w141 = FALSE ("Visible")
            w140 = FALSE ("Visible")
            n82 = property on="Motor" class="Clust (strict)"("Visible"=w140) -> ()  [unwired: 2 in, 2 out]
            n83 = property on="Test Ring" class="Ring (strict)"("Visible"=w140) -> ()  [unwired: 2 in, 2 out]
            n84 = property on="Rev/Fwd" class="Clust (strict)"("Visible"=w141) -> ()  [unwired: 2 in, 2 out]
            n85 = property on="On/Off" class="Bool (strict)"("Visible"=w141) -> ()  [unwired: 2 in, 2 out]
            n86 = property on="Test Slider" class="Slide (strict)"("Visible"=w141) -> ()  [unwired: 2 in, 2 out]
          }
          frame "Analog Out", "Motor", "PWM" {
            w147 = FALSE ("Visible")
            n87 = case shown="\"Analog Out\"" w146 {
              tunnel: [1.0 ("Value") -1.0 ("Value") 0.0 ("Value")] -> w145
              tunnel: [255.0 ("Value") 1.0 ("Value") 5.0 ("Value")] -> w144
              tunnel: [128.0 ("Value") 0.0 ("Value") 0.0 ("Value")] -> w143
              tunnel: [64.0 ("Value") 0.5 ("Value") 1.0 ("Value")] -> w142
              frame "PWM" {
              }
              frame "Motor", Default {
              }
              frame "Analog Out" {
              }
            }
            n88 = property on="Motor" class="Clust (strict)"("Visible"=TRUE) -> ()  [unwired: 2 in, 2 out]
            n89 = property on="Value" class="Slide (strict)"("Value"=w143, "Scale.Minimum"=w145, "Scale.Maximum"=w144, "Scale.Increment"=w142) -> ()  [unwired: 2 in, 2 out]
            n90 = property on="On/Off" class="Bool (strict)"("Visible"=w147) -> ()  [unwired: 2 in, 2 out]
            n91 = property on="Test Slider" class="Slide (strict)"("Visible"=w147) -> ()  [unwired: 2 in, 2 out]
            n92 = property on="Test Ring" class="Ring (strict)"("Visible"=w147) -> ()  [unwired: 2 in, 2 out]
            n93 = property on="Rev/Fwd" class="Clust (strict)"("Visible"=w147) -> ()  [unwired: 2 in, 2 out]
          }
          frame "Servo" {
            w163 = FALSE ("Visible")
            n94 = call <vilib>:"NT Read Number.vi"("name"=w165) -> ("value"=w164:dbl)  [unwired: 8 in, 2 out]
            n95 = property on="Test Slider" class="Slide (strict)"("Visible"=TRUE, "Scale.Maximum"=170.0 ("Scale.Range:Maximum")) -> ()  [unwired: 2 in, 2 out]
            n96 = local write "Test Slider"(w164) -> ()
            n97 = property on="Motor" class="Clust (strict)"("Visible"=w163) -> ()  [unwired: 2 in, 2 out]
            n98 = property on="Rev/Fwd" class="Clust (strict)"("Visible"=w163) -> ()  [unwired: 2 in, 2 out]
            n99 = property on="On/Off" class="Bool (strict)"("Visible"=w163) -> ()  [unwired: 2 in, 2 out]
            n100 = property on="Test Ring" class="Ring (strict)"("Visible"=w163) -> ()  [unwired: 2 in, 2 out]
          }
          frame "Relay", "Solenoid" {
            w166 = FALSE ("Visible")
            n101 = property on="Motor" class="Clust (strict)"("Visible"=w166) -> ()  [unwired: 2 in, 2 out]
            n102 = property on="Test Slider" class="Slide (strict)"("Visible"=w166) -> ()  [unwired: 2 in, 2 out]
            n103 = Search and Replace String(input string=w167, search string="/Value  **", replace string="/Direction") -> (result string=w173:string)  [unwired: 5 in, 3 out]
            n104 = property on="Test Ring" class="Ring (strict)"("Visible"=w166) -> ()  [unwired: 2 in, 2 out]
            n105 = call <vilib>:"NT Read String.vi"("name"=w173) -> ("value"=w171:string)  [unwired: 8 in, 2 out]
            n106 = Equal?(x="Both directions", y=w171) -> (x = y?=w169:bool)
            n107 = Not(x=w169) -> (.not. x?=w170:bool)
            n108 = property on="Rev/Fwd" class="Clust (strict)"("Visible"=w169) -> ()  [unwired: 2 in, 2 out]
            n109 = property on="On/Off" class="Bool (strict)"("Visible"=w170, "Caption.Text"=w168) -> ()  [unwired: 2 in, 2 out]
          }
          frame "Compressor", "Digital Out" {
            w176 = FALSE ("Visible")
            # "Get direction and finish"
            n110 = property on="Motor" class="Clust (strict)"("Visible"=w176) -> ()  [unwired: 2 in, 2 out]
            n111 = property on="Test Slider" class="Slide (strict)"("Visible"=w176) -> ()  [unwired: 2 in, 2 out]
            n112 = property on="Test Ring" class="Ring (strict)"("Visible"=w176) -> ()  [unwired: 2 in, 2 out]
            n113 = property on="On/Off" class="Bool (strict)"("Visible"=TRUE, "Caption.Text"=w177) -> ()  [unwired: 2 in, 2 out]
            n114 = property on="Rev/Fwd" class="Clust (strict)"("Visible"=FALSE) -> ()  [unwired: 2 in, 2 out]
          }
          frame "Camera" {
            n115 = call <vilib>:"NT_Get Last Path Segment.vi"("String in"=w184) -> ("String out"=w185:string)  [unwired: 10 in]
            n116 = property on="On/Off" class="Bool (strict)"("Visible"=FALSE) -> ()  [unwired: 2 in, 2 out]
            n117 = property on="Motor" class="Clust (strict)"("Visible"=FALSE) -> ()  [unwired: 2 in, 2 out]
            n118 = property on="Rev/Fwd" class="Clust (strict)"("Visible"=FALSE) -> ()  [unwired: 2 in, 2 out]
            n119 = case shown="\"White Balance  **\"" w185 {
              tunnel: w184 -> [w191 w200 w209 w218 w227 _ w233]
              tunnel: w183 -> [w189 w197 w206 w215 w224 _ _]
              frame "Size  **" {
                n120 = Index Array(array=w189) -> (element=w188:cluster{string[]})  [unwired: 1 in]
                n121 = call <vilib>:"NT Read String.vi"("name"=w191) -> ("value"=w190:string)  [unwired: 8 in, 2 out]
                n122 = Unbundle(w188) -> (w186:string[])
                n123 = Match First String(2:w186, 3:w190) -> (0:w187:i32)  [unwired: 1 out]
                n124 = property on="Test Ring" class="Ring (strict)"("Value"=w187, "Strings []"=w186) -> ()  [unwired: 2 in, 2 out]
                n125 = property on="Test Ring" class="Ring (strict)"("Visible"=TRUE) -> ()  [unwired: 2 in, 2 out]
                n126 = property on="Test Slider" class="Slide (strict)"("Visible"=FALSE) -> ()  [unwired: 2 in, 2 out]
              }
              frame "White Balance  **" {
                n127 = Index Array(array=w197, index=1) -> (element=w198:cluster{string[]})
                n128 = call <vilib>:"NT Read String.vi"("name"=w200) -> ("value"=w199:string)  [unwired: 8 in, 2 out]
                n129 = Unbundle(w198) -> (w195:string[])
                n130 = Match First String(2:w195, 3:w199) -> (0:w194:i32)  [unwired: 1 out]
                n131 = property on="Test Ring" class="Ring (strict)"("Value"=w194, "Strings []"=w195) -> ()  [unwired: 2 in, 2 out]
                n132 = property on="Test Ring" class="Ring (strict)"("Visible"=TRUE) -> ()  [unwired: 2 in, 2 out]
                n133 = property on="Test Slider" class="Slide (strict)"("Visible"=FALSE) -> ()  [unwired: 2 in, 2 out]
              }
              frame "Exposure  **" {
                n134 = Index Array(array=w206, index=2) -> (element=w207:cluster{string[]})
                n135 = call <vilib>:"NT Read String.vi"("name"=w209) -> ("value"=w208:string)  [unwired: 8 in, 2 out]
                n136 = Unbundle(w207) -> (w203:string[])
                n137 = Match First String(2:w203, 3:w208) -> (0:w204:i32)  [unwired: 1 out]
                n138 = property on="Test Ring" class="Ring (strict)"("Value"=w204, "Strings []"=w203) -> ()  [unwired: 2 in, 2 out]
                n139 = property on="Test Ring" class="Ring (strict)"("Visible"=TRUE) -> ()  [unwired: 2 in, 2 out]
                n140 = property on="Test Slider" class="Slide (strict)"("Visible"=FALSE) -> ()  [unwired: 2 in, 2 out]
              }
              frame "Exposure Priority  **" {
                n141 = Index Array(array=w215, index=3) -> (element=w216:cluster{string[]})
                n142 = call <vilib>:"NT Read String.vi"("name"=w218) -> ("value"=w217:string)  [unwired: 8 in, 2 out]
                n143 = Unbundle(w216) -> (w212:string[])
                n144 = Match First String(2:w212, 3:w217) -> (0:w213:i32)  [unwired: 1 out]
                n145 = property on="Test Ring" class="Ring (strict)"("Value"=w213, "Strings []"=w212) -> ()  [unwired: 2 in, 2 out]
                n146 = property on="Test Ring" class="Ring (strict)"("Visible"=TRUE) -> ()  [unwired: 2 in, 2 out]
                n147 = property on="Test Slider" class="Slide (strict)"("Visible"=FALSE) -> ()  [unwired: 2 in, 2 out]
              }
              frame "Color Enable  **" {
                n148 = Index Array(array=w224, index=4) -> (element=w225:cluster{string[]})
                n149 = call <vilib>:"NT Read String.vi"("name"=w227) -> ("value"=w226:string)  [unwired: 8 in, 2 out]
                n150 = Unbundle(w225) -> (w221:string[])
                n151 = Match First String(2:w221, 3:w226) -> (0:w222:i32)  [unwired: 1 out]
                n152 = property on="Test Ring" class="Ring (strict)"("Value"=w222, "Strings []"=w221) -> ()  [unwired: 2 in, 2 out]
                n153 = property on="Test Ring" class="Ring (strict)"("Visible"=TRUE) -> ()  [unwired: 2 in, 2 out]
                n154 = property on="Test Slider" class="Slide (strict)"("Visible"=FALSE) -> ()  [unwired: 2 in, 2 out]
              }
              frame Default {
                n155 = property on="Test Ring" class="Ring (strict)"("Visible"=FALSE) -> ()  [unwired: 2 in, 2 out]
                n156 = property on="Test Slider" class="Slide (strict)"("Visible"=FALSE) -> ()  [unwired: 2 in, 2 out]
              }
              frame "Brightness  **", "Color Level  **", "Compression  **", "FPS  **", "Sharpness  **" {
                n157 = call <vilib>:"NT Read Number.vi"("name"=w233) -> ("value"=w232:dbl)  [unwired: 8 in, 2 out]
                n158 = local write "Test Slider"(w232) -> ()
                n159 = property on="Test Ring" class="Ring (strict)"("Visible"=FALSE) -> ()  [unwired: 2 in, 2 out]
                n160 = property on="Test Slider" class="Slide (strict)"("Visible"=TRUE, "Scale.Maximum"=100.0 ("Scale.Range:Maximum")) -> ()  [unwired: 2 in, 2 out]
              }
            }
          }
        }
        n161 = property on="Progress" class="Clust (strict)"("Visible"=FALSE) -> ()  [unwired: 2 in, 2 out]
      }
      event "Test Name": Mouse Enter {
        # "Populate the ring with the list of tests"
        n162 = event-data() -> ()  [unwired: 1 in, 1 out]
        n163 = call <vilib>:"NT Read String Array.vi"("name"="TestMode/TestList" ("Name")) -> ("value"=w240:string[])  [unwired: 8 in, 2 out]
        n164 = Build Array (concatenate)("Select the test to run...", w240) -> (w239:string[])
        n165 = property on="Test Name" class="Ring (strict)"("Strings []"=w239) -> ()  [unwired: 2 in, 2 out]
      }
      event "Test Name": Value Change {
        w241 = FALSE ("Visible")
        # "Tell the robot the test name to run"
        n166 = event-data() -> ("NewVal"=w245:u16)  [unwired: 1 in]
        n167 = property on="Test Name" class="Ring (strict)"() -> ("Strings []"=w246:string[])  [unwired: 2 in, 2 out]
        n168 = local write "Progress"(T6 {"Test Progress"=0, "Test Progress Text"=""} ("Progress")) -> ()
        n169 = Index Array(array=w246, index=w245) -> (element=w244:string)
        n170 = call <vilib>:"NT Write String.vi"("value"=w244, "name"="TestMode/TestName" ("Name")) -> ()  [unwired: 9 in, 1 out]
        n171 = property on="Progress" class="Clust (strict)"("Visible"=TRUE) -> ()  [unwired: 2 in, 2 out]
        n172 = property on="Motor" class="Clust (strict)"("Visible"=w241) -> ()  [unwired: 2 in, 2 out]
        n173 = property on="Test Slider" class="Slide (strict)"("Visible"=w241) -> ()  [unwired: 2 in, 2 out]
        n174 = property on="On/Off" class="Bool (strict)"("Visible"=w241) -> ()  [unwired: 2 in, 2 out]
        n175 = property on="Rev/Fwd" class="Clust (strict)"("Visible"=w241) -> ()  [unwired: 2 in, 2 out]
        n176 = property on="Test Ring" class="Ring (strict)"("Visible"=w241) -> ()  [unwired: 2 in, 2 out]
      }
      event "Select Auto": Mouse Enter {
        # "Populate the combo box with the list of autonomous options"
        n177 = event-data() -> ()  [unwired: 1 in, 1 out]
        n178 = call <vilib>:"NT Read String Array.vi"("name"="Auto List" ("Name")) -> ("value"=w248:string[])  [unwired: 8 in, 2 out]
        n179 = property on="Select Auto" class="CmbBox"("Strings[]"=w248) -> ()  [unwired: 2 in, 2 out]
      }
      event "Select Auto": Value Change {
        # "User modified the Auto Selection. Write to NT variable so robot knows."
        n180 = event-data() -> ("NewVal"=w250:string)  [unwired: 1 in]
        n181 = call <vilib>:"NT Write String.vi"("value"=w250, "name"="Auto Selector" ("Name")) -> ()  [unwired: 9 in, 1 out]
      }
      event "CheckList": Double Click {
        # "Shift clears all"
        # "Update symbols on the listbox"
        n182 = event-data() -> ("PlatMods.Shift"=w252:bool, "Row"=w254:i32)  [unwired: 1 in]
        n183 = case shown="True" w252 {
          tunnel: w254 -> [w258 _]
          tunnel: 1 -> [w257 _]
          frame False {
            n184 = property on="CheckList" class="LstBox (strict)"() -> ("Item Symbols"=w256:i32[])  [unwired: 2 in, 2 out]
            n185 = Replace Array Subset(array=w256, new element=w257, index=w258) -> (w255:i32[])
            n186 = property on="CheckList" class="LstBox (strict)"("Item Symbols"=w255) -> ()  [unwired: 2 in, 2 out]
          }
          frame True {
            w259 = 0 ("Top Row")
            n187 = property on="CheckList" class="LstBox (strict)"() -> ("Number of Rows"=w261:u32)  [unwired: 2 in, 2 out]
            n188 = Initialize Array(0, w261) -> (w260:i32[])
            n189 = property on="CheckList" class="LstBox (strict)"("Top Row"=w259, "Value"=w259, "Item Symbols"=w260) -> ()  [unwired: 2 in, 2 out]
          }
        }
      }
      event "CheckList": Key Down {
        # "Update symbols on the listbox\nLeft and right keys check and uncheck"
        n190 = event-data() -> ("VKey"=w264:T18)  [unwired: 1 in]
        n191 = case shown="\"Left\", \"Right\"" w264 {
          selector: w264 -> [w269 _]
          tunnel: eventvkey."Left" ("VKey") -> [w267 _]
          frame "Left", "Right" {
            n192 = Equal?(x=w267, y=w269) -> (x = y?=w268:bool)
            n193 = Select(t=0, s=w268, f=1) -> (s? t:f=w270:i32)
            n194 = property on="CheckList" class="LstBox (strict)"() -> ("Item Symbols"=w273:i32[])  [unwired: 2 in, 2 out]
            n195 = Replace Array Subset(array=w273, new element=w270, index="CheckList") -> (w272:i32[])
            n196 = property on="CheckList" class="LstBox (strict)"("Item Symbols"=w272) -> ()  [unwired: 2 in, 2 out]
          }
          frame Default {
          }
        }
      }
      event "Motor.Enable": Value Change {
        # "When the test mode otor enable helper is set, update that\ntree row item's value"
        n197 = event-data() -> ("NewVal"=w278:bool)  [unwired: 1 in]
        n198 = Unbundle("Motor") -> ("Value"=w277:dbl)  [unwired: 1 out]
        n199 = Select(t=w277, s=w278, f=0.0) -> (s? t:f=w275:dbl)
        n200 = call <vilib>:"NT Write Number.vi"("value"=w275, "name"=w274) -> ()  [unwired: 9 in, 1 out]
      }
      event "Test Slider": Value Change {
        # "When the test mode slider helper is set, update that\ntree row item's value"
        n201 = event-data() -> ("NewVal"=w280:dbl)  [unwired: 1 in]
        n202 = call <vilib>:"NT Write Number.vi"("value"=w280, "name"=w281) -> ()  [unwired: 9 in, 1 out]
      }
      event "On/Off": Value Change {
        # "When the test mode on/off helper value is set, update that\ntree row item's value"
        n203 = event-data() -> ("NewVal"=w284:bool)  [unwired: 1 in]
        n204 = Boolean To (0,1)(Boolean=w284) -> (0, 1=w283:i16)
        n205 = call <vilib>:"NT Write Number.vi"("value"=w283, "name"=w282) -> ()  [unwired: 9 in, 1 out]
      }
      event "Rev/Fwd": Value Change {
        # "When the test mode helper value for relays is set, update that\ntree row item's value"
        n206 = event-data() -> ("NewVal.Forward"=w291:bool, "NewVal.Reverse"=w290:bool)  [unwired: 1 in]
        n207 = Boolean To (0,1)(Boolean=w291) -> (0, 1=w287:i16)
        n208 = Boolean To (0,1)(Boolean=w290) -> (0, 1=w289:i16)
        n209 = Negate(x=w289) -> (-x=w288:i16)
        n210 = Add(x=w287, y=w288) -> (x+y=w286:i16)
        n211 = call <vilib>:"NT Write Number.vi"("value"=w286, "name"=w285) -> ()  [unwired: 9 in, 1 out]
      }
      event "Test Ring": Value Change {
        # "When a test mode helper value is selected from the ring,\nset the tree item's variable to the string value"
        n212 = event-data() -> ("NewVal"=w294:u16)  [unwired: 1 in]
        n213 = property on="Test Ring" class="Ring (strict)"() -> ("Strings []"=w295:string[])  [unwired: 2 in, 2 out]
        n214 = Index Array(array=w295, index=w294) -> (element=w293:string)
        n215 = call <vilib>:"NT Write String.vi"("value"=w293, "name"=w292) -> ()  [unwired: 9 in, 1 out]
      }
      event "Rec Mode": Value Change {
        # "Update globals for recording mode and path to read log from.\nClear when logging and let NetworkTables set path for vision to\nuse."
        n216 = event-data() -> ("NewVal"=w302:enum32{"Stop", "Record", "Playback"})  [unwired: 1 in]
        n217 = global write "WPI_DashboardLogging Global.vi" "Logging Filename"(path "") -> ()
        n218 = global write "WPI_DashboardLogging Global.vi" "Recording"(w302) -> ()
        n219 = case shown="\"Playback\"" w302 {
          tunnel: w301 -> [_ w304 w312]
          tunnel: [_ _ w311] -> w299
          tunnel: [_ _ w310] -> _
          tunnel: w297 -> [_ _ w308]
          tunnel: cluster{i32, i32} {-250, 170} -> [_ _ w307]
          tunnel: [_ _ T19 {"Image Size"=TRUE, "Image Type"=TRUE, "Pixel Value"=TRUE, "ROI Information"=TRUE, "Zoom Factor"=FALSE} ("Image Information Shown:All Elements")] -> _
          tunnel: [_ _ TRUE ("Zoom Factor")] -> _
          frame Default {
          }
          frame "Stop", "Record" {
            # "Place Window too"
            n220 = invoke class="VI" method="FP.Close"(reference=w304) -> (reference out=w303:refnum<vi>)  [unwired: 2 in, 2 out]
            n221 = invoke class="VI" method="Abort VI"(reference=w303) -> ()  [unwired: 2 in, 3 out]
          }
          frame "Playback" {
            n222 = call "Open Playback Panel.vi"("Offset"=w307, "DB VI Ref"=w308, "Playback in"=w312) -> ("Playback out"=w309:refnum<vi>)  [unwired: 8 in]
            n223 = register-events(w309) -> (reference out=w311:refnum<event-registration>, error out=w310:errorcluster)  [unwired: 2 in]
          }
        }
        n224 = call <vilib>:"WPI_DashboardNT Log FieldName Cache.vi"("Operation"=enum16{"Lookup/Add", "Index", "Clear"}."Clear") -> ()  [unwired: 8 in, 3 out]
      }
      event Panel Close {
        w313 = enum32{"Stop", "Record", "Playback"}."Stop" ("Rec Mode")
        # "Playback window has been closed, abort"
        n225 = event-data() -> ()  [unwired: 1 in, 4 out]
        n226 = local write "Rec Mode"(w313) -> ()
        n227 = global write "WPI_DashboardLogging Global.vi" "Recording"(w313) -> ()
      }
      event Panel Close {
        # "Abort playback window and ourself"
        n228 = event-data() -> ()  [unwired: 1 in, 4 out]
        n229 = invoke class="VI" method="FP.Close"(reference=w319) -> (reference out=w318:refnum<vi>)  [unwired: 2 in, 2 out]
        n230 = invoke class="VI" method="FP.Close"(reference=w314) -> (reference out=w316:refnum<vi>)  [unwired: 2 in, 2 out]
        n231 = invoke class="VI" method="Abort VI"(reference=w318) -> (error out=w317:errorcluster)  [unwired: 2 in, 2 out]
        n232 = invoke class="VI" method="Abort VI"(reference=w316) -> (error out=w315:errorcluster)  [unwired: 2 in, 2 out]
        n233 = invoke class="VI" method="Abort VI"(error in=w317) -> ()  [unwired: 2 in, 3 out]
        n234 = invoke class="VI" method="Abort VI"(error in=w315) -> ()  [unwired: 2 in, 3 out]
      }
      event "Tree": Double Click {
        n235 = event-data() -> ("PlatMods"=w325:T21, "Tag"=w322:string)  [unwired: 1 in]
        n236 = Unbundle(w325) -> ("Shift"=w324:bool)  [unwired: 4 out]
        n237 = String Subset(string=w322, length (rest)=1 ("length (rest)")) -> (substring=w321:string)  [unwired: 1 in]
        n238 = Not(x=w324) -> (.not. x?=w323:bool)
        n239 = case shown="\"/\"" w321 {
          tunnel: w322 -> [_ w327]
          tunnel: w323 -> [_ w326]
          frame Default {
          }
          frame "/" {
            n240 = call <vilib>:"NT Update Persistence.vi"("Persistence"=w326, "Name"=w327) -> ()  [unwired: 9 in, 1 out]
          }
        }
      }
    }
  }
  n241 = while {
    tunnel: w46 -> [w330]
    i -> [w332]
    stop <- FALSE stop-if-true
    n242 = Wait (ms)(milliseconds to wait=u32 100) -> ()  [unwired: 1 out]
    n243 = case shown="\"Playback\"" "Rec Mode" {
      tunnel: w332 -> [_ _ w347]
      tunnel: [u32 2829099 ("Base Color") u32 11141120 ("Target Color") w336] -> w329
      frame "Stop", Default {
        # "Reset the color, extra updates don't cost much"
      }
      frame "Record" {
      }
      frame "Playback" {
        # "Playback"
        n244 = Quotient & Remainder(x=w347, y=u32 50 ("milliseconds to wait")) -> (x-y*floor(x/y)=w343:u32)  [unwired: 1 out]
        n245 = Divide(x=w343, y=u32 50 ("milliseconds to wait")) -> (x/y=w340:dbl)
        n246 = Multiply(x=6.283185307179586, y=w340) -> (x*y=w345:dbl)
        n247 = Sine(x=w345) -> (sin(x)=w344:dbl)
        n248 = Absolute Value(x=w344) -> (abs(x)=w337:dbl)
        n249 = call "Interpolate RGB Color.vi"("Proportion"=w337, "Target Color"=u32 30976, "Base Color"=u32 2829099) -> ("Result Color"=w336:u32)  [unwired: 8 in]
      }
    }
    n250 = global write "DashBoardGlobals.vi" "Rec Mode"("Rec Mode") -> ()
    n251 = property class="Pane"(reference=w330, "PaneColor"=w329) -> ()  [unwired: 1 in, 2 out]
  }
  n252 = local write "Dashboard Tab"(T2."Custom" ("Dashboard Tab")) -> ()
  n253 = property on="On/Off" class="Bool (strict)"("Visible"=w19) -> ()  [unwired: 2 in, 2 out]
  n254 = property on="Motor" class="Clust (strict)"("Visible"=w19) -> ()  [unwired: 2 in, 2 out]
  n255 = property on="Progress" class="Clust (strict)"("Visible"=w19) -> ()  [unwired: 2 in, 2 out]
  n256 = property on="Test Ring" class="Ring (strict)"("Visible"=w19) -> ()  [unwired: 2 in, 2 out]
  n257 = property on="Rev/Fwd" class="Clust (strict)"("Visible"=w19) -> ()  [unwired: 2 in, 2 out]
  n258 = while {
    tunnel: u16 1741 ("timeout ms (25000)") -> [w349]
    stop <- FALSE stop-if-true
    n259 = TCP Create Listener(10:w349) -> (0:w348:errorcluster, 3:w350:refnum<k5>)  [unwired: 4 in, 1 out]
    n260 = case shown="No Error" w348 {
      selector: w348 -> [w352 _]
      tunnel: w350 -> [w353 _]
      frame No Error {
        n261 = while {
          tunnel: w353 -> [w356]
          tunnel: w352 -> [w355]
          stop <- FALSE stop-if-true
          n262 = TCP Wait On Listener(8:w355, 11:w356) -> (0:w357:errorcluster, 4:w358:refnum<k5>)  [unwired: 2 in, 3 out]
          n263 = local write "TCP"(w358) -> ()
          n264 = case shown="Error" w357 {
            frame No Error {
            }
            frame Error {
              n265 = Wait (ms)(milliseconds to wait=u32 1000) -> ()  [unwired: 1 out]
            }
          }
        }
      }
      frame Error {
        n266 = Wait (ms)(milliseconds to wait=u32 1000) -> ()  [unwired: 1 out]
      }
    }
  }
  n267 = global write "WPI_DashboardLogging Global.vi" "Recording"(w41) -> ()
  n268 = local write "Rec Mode"(w41) -> ()
  n269 = vi-ref "FieldDisplaySmall.vi"() -> (w10:refnum<vi>)
  n270 = call <vilib>:"NT Write String.vi"("value"="Select Auto", "name"="Auto Selector" ("Name")) -> ()  [unwired: 9 in, 1 out]
  n271 = invoke class="VI" method="Run VI"(reference=w10, "Wait until done"=FALSE ("Wait Until Done")) -> (reference out=w8:refnum<vi>)  [unwired: 3 in, 4 out]
  n272 = invoke on="FieldSubpanel" class="SubPnl" method="Insert VI"("VI Ref"=w8) -> ()  [unwired: 3 in, 4 out]
